vi "MI Sync with TClk (MAIN) repeatability.vi"(10 "FGENs":refnum<k15>[](array[refnum])=["FGEN1", "FGEN2"] caption="Resource Name", 11 "Scopes":refnum<k15>[](array[refnum])=["SCOPE1", "SCOPE2"] caption="resource name") -> (1 "Preparing T-Clk":bool, 2 "Waveform Graph":waveform(dbl)[](graph), 3 "relative trigger position (s)":dbl[](array[numeric]) format="%#.3p")   [LabVIEW 2024]
doc: "This VI is a one shot example of synchronising 2x arb with 2 and 1 channels with 2x scopes with 2 and 1 channel.\nThe frequency the arb are to produce is set on the front panel and all are identical amplitude and frequency with the phase set to a 120 degree difference.\nTriggering of the oscilloscope is based on channel 0 of the first specified scope module as the signal crosses zero."
uses:
  <vilib>/measure/NI_MAPro.lvlib
  <vilib>/Analysis/NI_AALBase.lvlib
  <vilib>/measure/matone.llb/Extract Single Tone Information N Chan.vi
  <instrlib>/niScope/Acquire/Fetch/niScope Multi Fetch WDT.vi
panel:
  out "Progress":dbl(slide) scale=0.0..100.0
  out "min relative trigger position":dbl format="%#_6p"
  out "max relative trigger position":dbl format="%#_6p"
  in  "Number of repeats":i32=1
  out "Histogram Graph Relative Trigger Positions":T1(graph)
  out "detected frequencies (Hz)":dbl[](array[numeric])
  out "detected phases (deg)":dbl[](array[numeric])
  # "Hardware Configuration"
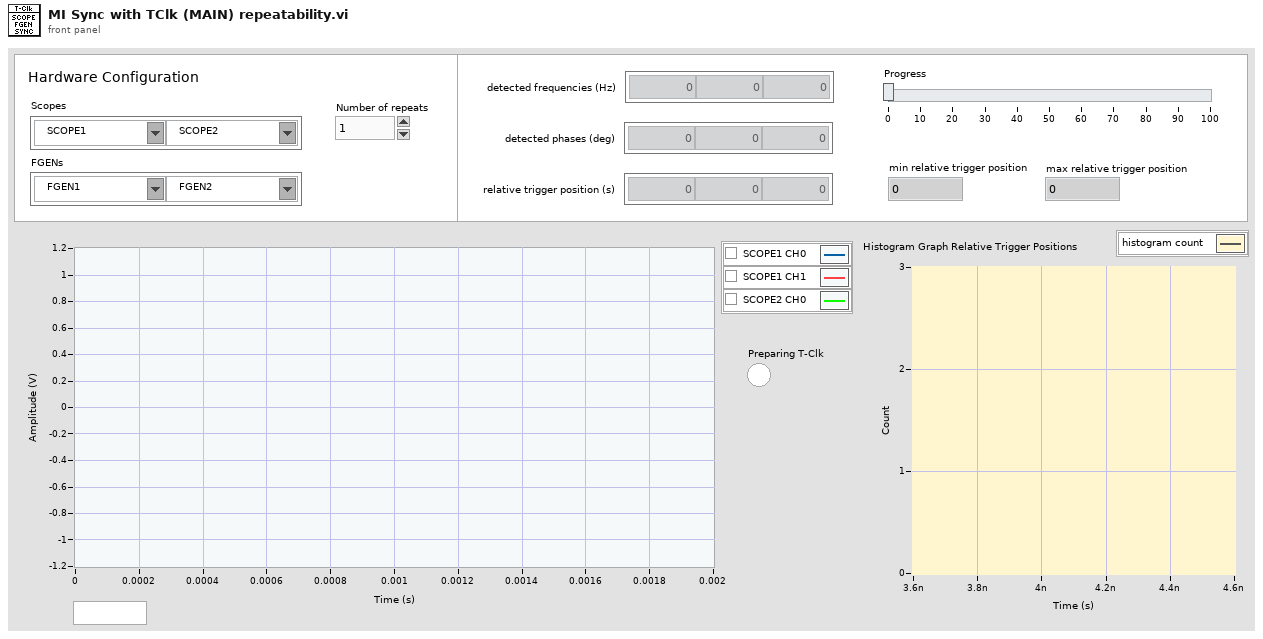
[diagram p1: front panel]
types:
  T1 = cluster{"X Values":dbl[], "Histogram: h(x)":i32[]}
  T2 = cluster{"actualSamples":i32, "absoluteInitialX":dbl, "relativeInitialX":dbl, "xIncrement":dbl, "offset":dbl, "gain":dbl, "reserved1":dbl, "reserved2":dbl}[]
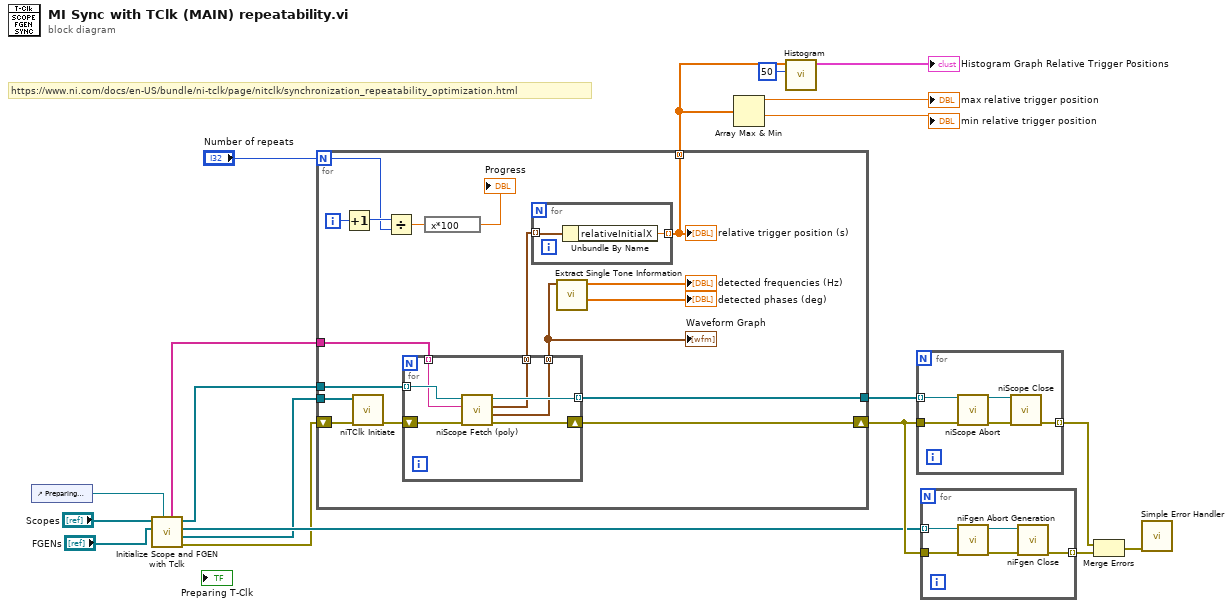
[diagram p0: block diagram]
diagram:
  # "https://www.ni.com/docs/en-US/bundle/ni-tclk/page/nitclk/synchronization_repeatability_optimization.html"
  n1 = control-ref of="Preparing T-Clk"() -> (w3:refnum<vi>)
  n2 = call "Initialize Scope and FGEN with Tclk.vi"("Tclk Boolean Ref"=w3, "FGEN Resources in"="FGENs", "Scope Resources in"="Scopes") -> ("error out"=w7:errorcluster, "Tclk Refs Array"=w5:refnum<k20>[], "FGEN Resources out"=w14:refnum<k15>[], "Scope Resources out"=w6:refnum<k15>[], "scope channels"=w4:string[])  [unwired: 4 in]
  n3 = for {
    N: "Number of repeats" -> [w24]
    tunnel: w5 -> [w36]
    tunnel: w6 -> [w34]
    tunnel: [w33] -> w19
    tunnel: w4 -> [w31]
    tunnel: [w27] -> w9 mode=concatenating
    shift-right: [w30] -> w16
    shift-left: w7 -> [w35]
    i -> [w26]
    n4 = Increment(x=w26) -> (x+1=w25:i32)
    n5 = call <instrlib>:"niTClk Initiate.vi"("error in (no error)"=w35, "sessions"=w36) -> ("error out"=w32:errorcluster)  [unwired: 8 in, 1 out]
    n6 = Divide(x=w25, y=w24) -> (x/y=w23:dbl)
    n7 = for {
      tunnel: w34 -> [w43] mode=indexing
      tunnel: [w42] -> w33 mode=indexing
      tunnel: [w39] -> w20 mode=concatenating
      tunnel: w31 -> [w38] mode=indexing
      tunnel: [w37] -> w28 mode=concatenating
      shift-right: [w41] -> w30
      shift-left: w32 -> [w40]
      n8 = call-poly <instrlib>:"niScope Fetch (poly).vi"("error in"=w40, "channels"=w38, "instrument handle"=w43) -> ("error out"=w41:errorcluster, "wfm"=w39:waveform(dbl)[], "wfm info"=w37:T2, "instrument handle out"=w42:refnum<k15>)  [unwired: 5 in]
    }
    "Waveform Graph" <- w20
    n9 = expression code="x*100"(w23) -> (→"Progress":dbl)
    n10 = for {
      tunnel: w28 -> [w45] mode=indexing
      tunnel: [w44] -> w27 mode=indexing
      n11 = Unbundle By Name(w45) -> ("relativeInitialX"=w44:dbl)
    }
    "relative trigger position (s)" <- w27
    n12 = call-poly <vilib>:"Extract Single Tone Information.vi"("time signals in"=w20) -> ("detected phases (deg)"=→"detected phases (deg)":dbl[], "detected frequencies"=→"detected frequencies (Hz)":dbl[])  [unwired: 5 in, 4 out]
  }
  n13 = Array Max & Min(array=w9) -> (max value=→"max relative trigger position":dbl, min value=→"min relative trigger position":dbl)  [unwired: 2 out]
  n14 = call <vilib>:"Histogram.vi"("intervals"=50, "X"=w9) -> ("Histogram Graph"=→"Histogram Graph Relative Trigger Positions":T1)  [unwired: 6 in, 3 out]
  n15 = for {
    tunnel: w19 -> [w50] mode=indexing
    tunnel: w16 -> [w49]
    tunnel: [w48] -> w17 mode=indexing
    n16 = call <instrlib>:"niScope Abort.vi"("instrument handle"=w50, "error in"=w49) -> ("instrument handle out"=w47:refnum<k15>, "error out"=w46:errorcluster)  [unwired: 12 in]
    n17 = call <instrlib>:"niScope Close.vi"("instrument handle"=w47, "error in"=w46) -> ("error out"=w48:errorcluster)  [unwired: 13 in]
  }
  n18 = for {
    tunnel: w14 -> [w55] mode=indexing
    tunnel: [w54] -> w18 mode=indexing
    tunnel: w16 -> [w53]
    n19 = call <instrlib>:"niFgen Abort Generation.vi"("error in (no error)"=w53, "Instrument Handle"=w55) -> ("error out"=w52:errorcluster, "Instrument Handle Out"=w51:refnum<k15>)  [unwired: 8 in]
    n20 = call <instrlib>:"niFgen Close.vi"("error in (no error)"=w52, "Instrument Handle"=w51) -> ("error out"=w54:errorcluster)  [unwired: 9 in]
  }
  n21 = Merge Errors(w17, w18) -> (w15:errorcluster)
  n22 = call <vilib>:"Simple Error Handler.vi"("error in (no error)"=w15) -> ()  [unwired: 4 in, 5 out]
